vi "GetFreeRanges.vi"(8 "ErrorIn":errorcluster caption="Error In(no Error)", 9 "RequestedSize":i32, 11 "ReferenceIn":refnum<class "ErrorDefinitionSQLite.lvclass"> caption="Reference In") -> (0 "ErrorOut":errorcluster caption="Error Out", 1 "UsedSlots":cluster{"Size":i32, "StartOfNewRange":i32}[](array[cluster]), 2 "SlotsAvailable":cluster{"Size":i32, "StartOfNewRange":i32}[](array[cluster]), 3 "ReferenceOut":refnum<class "ErrorDefinitionSQLite.lvclass"> caption="Reference Out")   [LabVIEW 2018, in "ErrorDefinitionSQLite.lvclass"]
uses:
  ErrorDefinitionSQLite.lvclass
  <vilib>/drjdpowell/SQLite Library/SQL Connection/Execute SQL.vi
  <vilib>/drjdpowell/SQLite Library/SQLite.lvlib
  <vilib>/drjdpowell/SQLite Library/SQL Connection/Connection.lvclass
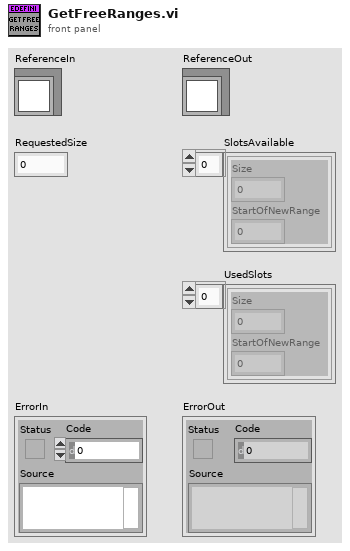
[diagram p1: front panel]
types:
  T1 = typedef "ErrorDefinitionSQLite.lvclass/ObjectAttributes.ctl" = cluster{"Path":path, "SQLiteRef":refnum<class "Connection.lvclass">, "EndOfRange":i32, "DefaultLibrarySize":i32, "StartOfRange":i32}
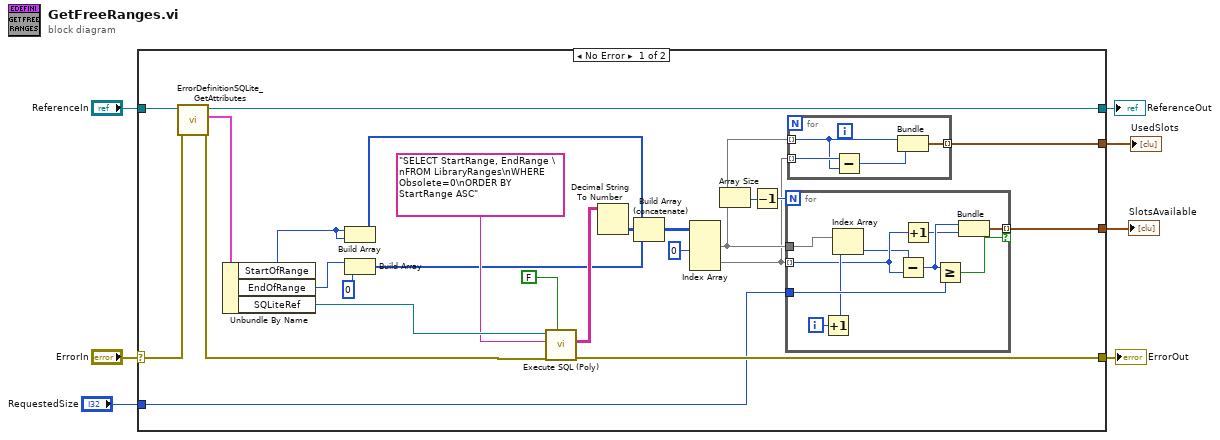
[diagram p0: block diagram]
diagram:
  n1 = case shown="No Error" "ErrorIn" {
    selector: "ErrorIn" -> [w32 w48]
    tunnel: [w26 w48] -> w6
    tunnel: [w30 w47] -> w4
    tunnel: "ReferenceIn" -> [w31 w47]
    tunnel: "RequestedSize" -> [w20 _]
    tunnel: [w13 _] -> w2
    tunnel: [w8 _] -> w1
    frame No Error {
      n2 = call "ErrorDefinitionSQLite_GetAttributes.vi"("ErrorIn"=w32, "Reference in"=w31) -> ("ErrorOut"=w21:errorcluster, "Data"=w29:T1, "Reference out"=w30:refnum<class "ErrorDefinitionSQLite.lvclass">)  [unwired: 6 in, 1 out]
      n3 = Unbundle By Name(w29) -> ("StartOfRange"=w12:i32, "EndOfRange"=w18:i32, "SQLiteRef"=w27:refnum<class "Connection.lvclass">)
      n4 = Build Array(w12, w12) -> (w11:i32[])
      n5 = Build Array(w18, 0 ("element")) -> (w16:i32[])
      n6 = call-poly <vilib>:"Execute SQL (Poly).vi"("Use SAVEPOINT"=FALSE, "error in (no error)"=w21, "SQL"="SELECT StartRange, EndRange \nFROM LibraryRanges\nWHERE Obsolete=0\nORDER BY StartRange ASC", "SQLite Connection in"=w27) -> ("error out"=w26:errorcluster, "Result Set"=w25:string[][])  [unwired: 4 in, 2 out]
      n7 = Decimal String To Number(string=w25) -> (number=w24:i32[][])  [unwired: 2 in, 1 out]
      n8 = Build Array (concatenate)(w11, w24, w16) -> (w19:i32[][])
      n9 = Index Array(array=w19, index (col) #1=0 ("disabled index (col)")) -> (element #1=w10:i32[], element #2=w9:i32[])  [unwired: 3 in]
      n10 = Array Size(array=w10) -> (size(s)=w15:i32)
      n11 = Decrement(x=w15) -> (x-1=w14:i32)
      n12 = for {
        N: w14 -> [_]
        tunnel: w10 -> [w38]
        tunnel: w9 -> [w39] mode=indexing
        tunnel: w20 -> [w46]
        tunnel: [w44] -> w13 mode=indexing if=w43
        i -> [w45]
        n13 = Increment(x=w45) -> (x+1=w40:i32)
        n14 = Index Array(array=w38, index=w40) -> (element=w37:i32)
        n15 = Subtract(x=w37, y=w39) -> (x-y=w42:i32)
        n16 = Increment(x=w39) -> (x+1=w41:i32)
        n17 = Greater Or Equal?(x=w42, y=w46) -> (x >= y?=w43:bool)
        n18 = Bundle(w42, w41) -> (w44:cluster{i32, i32})  [unwired: 1 in]
      }
      n19 = for {
        tunnel: w10 -> [w35] mode=indexing
        tunnel: w9 -> [w36] mode=indexing
        tunnel: [w33] -> w8 mode=indexing
        n20 = Subtract(x=w36, y=w35) -> (x-y=w34:i32)
        n21 = Bundle("element"=w35, w34) -> (w33:cluster{"element":i32, i32})  [unwired: 1 in]
      }
    }
    frame Error {
    }
  }
  "ErrorOut" <- w6
  "ReferenceOut" <- w4
  "SlotsAvailable" <- w2
  "UsedSlots" <- w1
